vi "check if above threshold.vi"(8 "error in (no error)":errorcluster, 11 "Autofocus in":refnum<class "Autofocus.lvclass">) -> (0 "error out":errorcluster, 3 "Autofocus out":refnum<class "Autofocus.lvclass">)   [LabVIEW 2012, in "Autofocus.lvclass"]
uses:
  Autofocus.lvclass
  Autofocus.lvclass/Autofocus.ctl
  <vilib>/Analysis/baseanly.llb/Mean (DBL).vi
  <vilib>/Analysis/NI_AALBase.lvlib
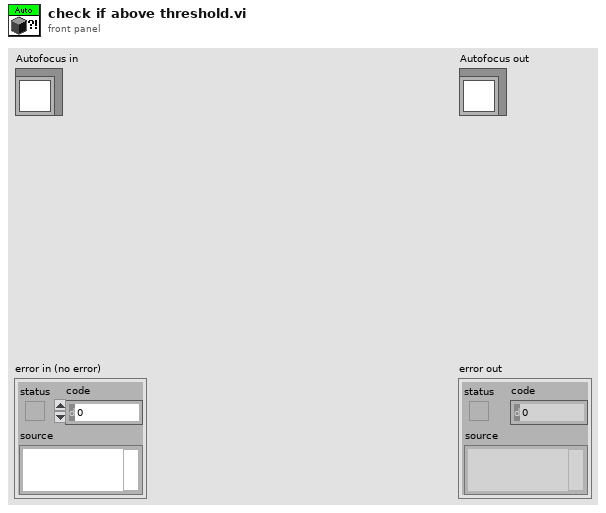
[diagram p1: front panel]
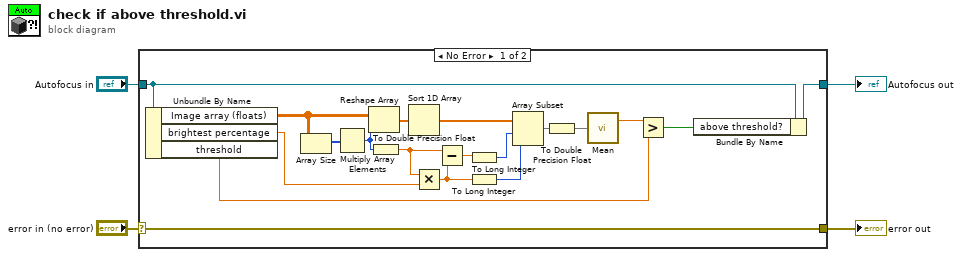
[diagram p0: block diagram]
diagram:
  n1 = case shown="No Error" "error in (no error)" {
    selector: "error in (no error)" -> [w23 w25]
    tunnel: [w23 w25] -> w3
    tunnel: [w8 w24] -> w1
    tunnel: "Autofocus in" -> [w9 w24]
    frame No Error {
      n2 = Unbundle By Name(w9) -> ("Image array (floats)"=w21:dbl[][], "brightest percentage"=w5:dbl, "threshold"=w6:dbl)
      n3 = Array Size(array=w21) -> (size(s)=w22:i32[])
      n4 = Multiply Array Elements(1:w22) -> (0:w16:i32)
      n5 = Reshape Array(w21, w16) -> (w20:dbl[])
      n6 = To Double Precision Float(number=w16) -> (double precision float=w14:dbl)
      n7 = Sort 1D Array(array=w20) -> (sorted array=w19:dbl[])
      n8 = Multiply(x=w14, y=w5) -> (x*y=w15:dbl)
      n9 = Subtract(x=w14, y=w15) -> (x-y=w12:dbl)
      n10 = To Long Integer(number=w12) -> (32bit integer=w11:i32)
      n11 = To Long Integer(number=w15) -> (32bit integer=w13:i32)
      n12 = Array Subset(array=w19, index=w11, length=w13) -> (w18:dbl[])
      n13 = To Double Precision Float(number=w18) -> (double precision float=w17:dbl[])
      n14 = call-poly <vilib>:"Mean.vi"("X"=w17) -> ("mean"=w10:dbl)  [unwired: 1 out]
      n15 = Greater?(x=w10, y=w6) -> (0:w7:bool)
      n16 = Bundle By Name(cluster=w9, "above threshold?"=w7) -> (w8:refnum<class "Autofocus.lvclass">)
    }
    frame Error {
    }
  }
  "error out" <- w3
  "Autofocus out" <- w1
